vi "例9.6 播放一首音乐快速VI.vi"() -> ()   [LabVIEW 2012]
doc: "本VI将直接播放声音文件并输出至扬声器。通过Play Sound File.vi打开文件并马上开始异步播放（相对于Sound File to Sound Output.vi范例中显示的方法）。"
panel:
  out "音乐波形":waveform(dbl)[](graph)
  in  "path":path caption="路径"
  in  "Device ID":u32 caption="设备ID" format="%.0x"
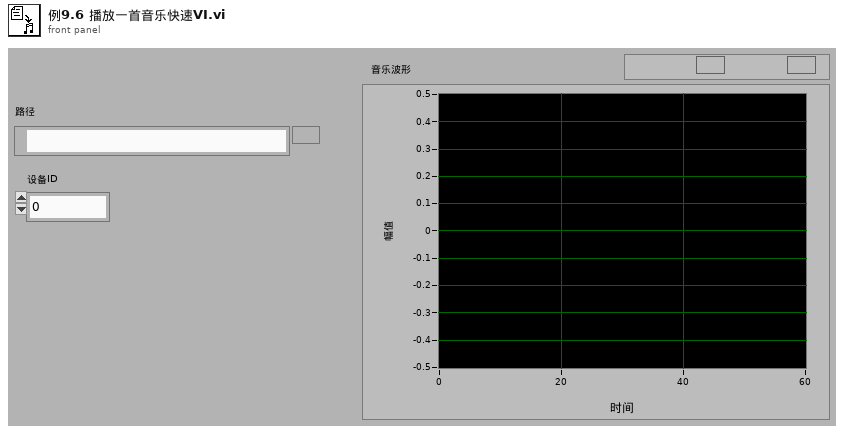
[diagram p1: front panel]
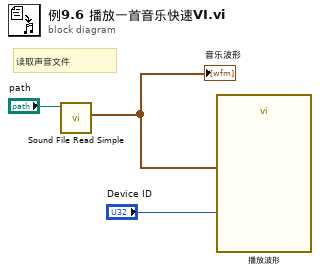
[diagram p0: block diagram]
diagram:
  # "读取声音文件"
  n1 = call <vilib>:"Sound File Read Simple.vi"("path"="path") -> ("data"=w2:waveform(dbl)[])  [unwired: 7 in, 3 out]
  "音乐波形" <- w2
  n2 = call "播放波形"("Device"="Device ID", "Data"=w2) -> ()  [unwired: 17 in, 1 out]
